vi "Read2 Channels Metodo.vi"(6 "Measurement Type (0: Phase)":i32(ring) items=["Phase", "Delay", "DelayRR", "DelayRF", "DelayFR", "DelayFF"], 8 "error in (no error)":errorcluster, 9 "Channels":T2={"Data Tektronix"={"Channel 1 (1: Channel 1)"=1, "Channel 2 (2: Channel 2)"=2}, "Data Keysight"={"Channels 2"=[], "Timeout (10000 ms)"=10000}} {"Data Keysight"."Channels 2" items=["Channel 1"=0, "Channel 2"=1, "Channel 3"=2, "Channel 4"=3, "Waveform Memory 1"=5, "Waveform Memory 2"=6, "Serial Bus 1"=7, "Serial Bus 2"=8, "Digital Bus Low"=9, "Digital Bus High "=10, "Digital Bus 1"=11, "Digital Bus 2"=12, "External"=29, "Function 1"=32, "Function 2"=33, "Function 3"=34, "Function 4"=35, "Math 1"=36, "Math 2"=37, "Math 3"=38, "Math 4"=39, "FFT"=40, "Analog Bus"=41]; "Data Tektronix"."Channel 2 (2: Channel 2)" items=["Channel 1"=1, "Channel 2"=2, "Channel 3"=3, "Channel 4"=4]; "Data Tektronix"."Channel 1 (1: Channel 1)" items=["Channel 1"=1, "Channel 2"=2, "Channel 3"=3, "Channel 4"=4]}, 11 "TektroniksTDS in":refnum<class "TektroniksTDS.lvclass">) -> (0 "error out":errorcluster, 1 "Data Out":T1, 3 "TektroniksTDS out":refnum<class "TektroniksTDS.lvclass">)   [LabVIEW 2020, in "TektroniksTDS.lvclass"]
uses:
  TektroniksTDS.lvclass
  TektroniksTDS.lvclass/TektroniksTDS.ctl
  <instrlib>/Tektronix TDS 200 1000 2000 Series/Tektronix TDS 200 1000 2000 Series.lvlib
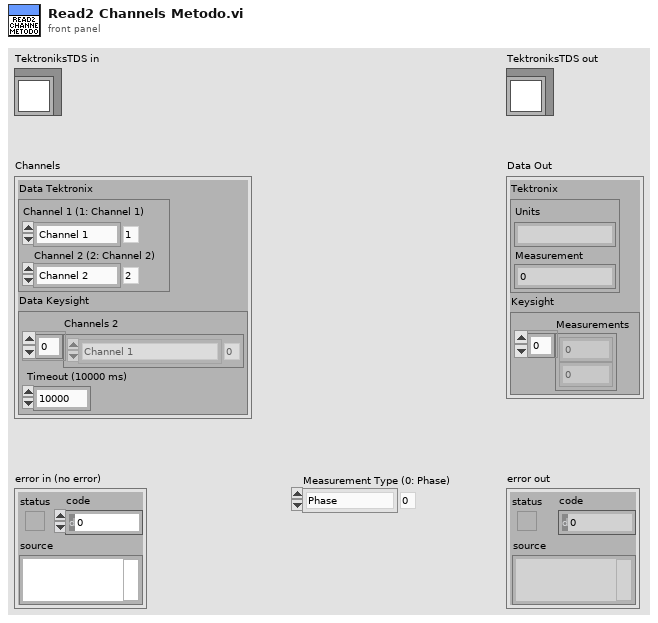
[diagram p1: front panel]
types:
  T1 = cluster{"Tektronix":cluster{"Units":string, "Measurement":dbl}, "Keysight":cluster{"Measurements":dbl[]}}
  T2 = cluster{"Data Tektronix":cluster{"Channel 1 (1: Channel 1)":i32, "Channel 2 (2: Channel 2)":i32}, "Data Keysight":cluster{"Channels 2":i32[], "Timeout (10000 ms)":u32}}
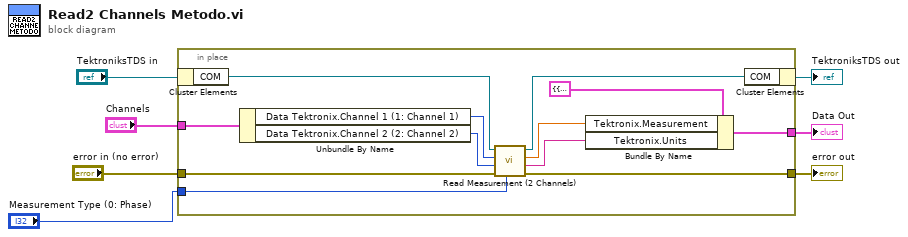
[diagram p0: block diagram]
diagram:
  n1 = in-place {
    in-place-border: "Measurement Type (0: Phase)" -> [w17]
    in-place-border: "Channels" -> [w16]
    in-place-border: "error in (no error)" -> [w13]
    in-place-border: [w12] -> w3
    in-place-border: [w9] -> w1
    n2 = in-place-cluster #1("TektroniksTDS in") -> ("COM"=w18:refnum<visa-resource-name>)
    n3 = Unbundle By Name(w16) -> ("Data Tektronix.Channel 1 (1: Channel 1)"=w15:i32, "Data Tektronix.Channel 2 (2: Channel 2)"=w14:i32)
    n4 = call <instrlib>:"Read Measurement (2 Channels).vi"("Measurement Type (0: Phase)"=w17, "error in (no error)"=w13, "Channel 2 (2: Channel 2)"=w14, "Channel 1 (1: Channel 1)"=w15, "VISA resource name"=w18) -> ("error out"=w12:errorcluster, "Units"=w10:string, "Measurement"=w11:dbl, "VISA resource name out"=w19:refnum<visa-resource-name>)  [unwired: 3 in]
    n5 = Bundle By Name(cluster=T1 {"Tektronix"={"Units"="", "Measurement"=0.0}, "Keysight"={"Measurements"=[]}} ("Data Out"), "Tektronix.Measurement"=w11, "Tektronix.Units"=w10) -> (w9:T1)
    n6 = in-place-cluster #1("COM"=w19) -> (→"TektroniksTDS out":refnum<class "TektroniksTDS.lvclass">)
  }
  "error out" <- w3
  "Data Out" <- w1
